vi "ParseArgumentsCore.vi"(8 "error in (no error)":errorcluster, 10 "Inputs":string[](array[string]), 11 "ExecuteBuildSpec in":refnum<class "ExecuteBuildSpec.lvclass">) -> (0 "error out":errorcluster, 3 "ExecuteBuildSpec out":refnum<class "ExecuteBuildSpec.lvclass">)   [LabVIEW 2014, in "ExecuteBuildSpec.lvclass"]
uses:
  ExecuteBuildSpec.lvclass
  ExecuteBuildSpec.lvclass/ExecuteBuildSpec.ctl
  Utilities/OperationErrorType.ctl
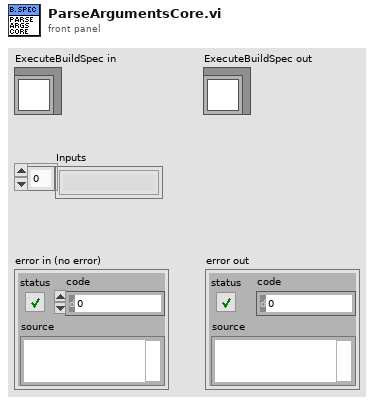
[diagram p1: front panel]
types:
  T1 = typedef "OperationErrorType.ctl" = enum16{"RequiredArgumentMissing", "UnknownArguments", "LoggerSetMultipleTimes", "OperationBrokenError"}
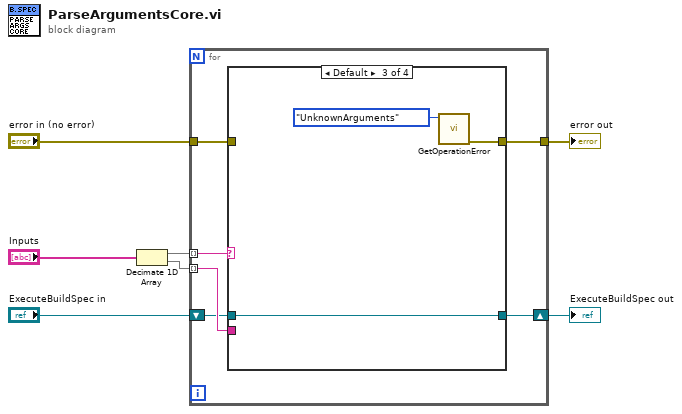
[diagram p0: block diagram]
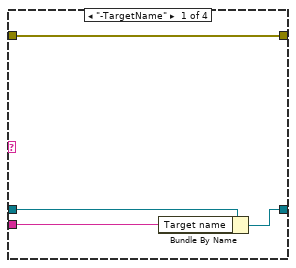
[diagram p2: hidden frame]
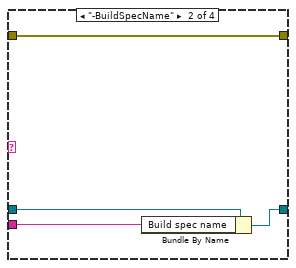
[diagram p3: hidden frame]
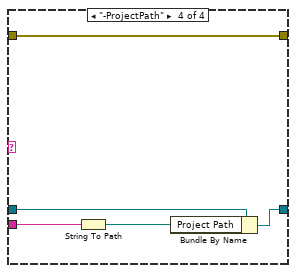
[diagram p4: hidden frame]
diagram:
  n1 = Decimate 1D Array("Inputs") -> (w2:string[], w3:string[])
  n2 = for {
    tunnel: w2 -> [w13] mode=indexing
    tunnel: w3 -> [w12] mode=indexing
    shift-right: [w10] -> w5
    shift-left: "ExecuteBuildSpec in" -> [w11]
    tunnel: "error in (no error)" -> [w9]
    tunnel: [w8] -> w7
    n3 = case shown="Default" w13 {
      tunnel: w12 -> [w14 w19 _ w28]
      tunnel: w11 -> [w17 w21 w24 w29]
      tunnel: [w16 w20 w24 w26] -> w10
      tunnel: w9 -> [w15 w18 _ w25]
      tunnel: [w15 w18 w23 w25] -> w8
      frame "-TargetName" {
        n4 = Bundle By Name(cluster=w17, "Target name"=w14) -> (w16:refnum<class "ExecuteBuildSpec.lvclass">)
      }
      frame "-BuildSpecName" {
        n5 = Bundle By Name(cluster=w21, "Build spec name"=w19) -> (w20:refnum<class "ExecuteBuildSpec.lvclass">)
      }
      frame Default {
        n6 = call "GetOperationError.vi"("Operation Error Type"=OperationErrorType."UnknownArguments") -> ("error out"=w23:errorcluster)  [unwired: 10 in]
      }
      frame "-ProjectPath" {
        n7 = String To Path(string=w28) -> (path=w27:path)
        n8 = Bundle By Name(cluster=w29, "Project Path"=w27) -> (w26:refnum<class "ExecuteBuildSpec.lvclass">)
      }
    }
  }
  "error out" <- w7
  "ExecuteBuildSpec out" <- w5
